vi "Write Channel.vi"(8 "error in (no error)":errorcluster, 10 "Channel":T1={"Coupling"=0, "Differential Input"=FALSE, "Direct-to-ADC"=FALSE, "Range"=2000, "Impedance"=50, "DC Offset"=0, "Filter"=0} {"Impedance" min=50 max=1000000 step=999950; "Coupling" items=["DC", "AC"]}, 11 "Initialize_card in":refnum<class "Control_card.lvclass">) -> (0 "error out":errorcluster, 3 "Initialize_card out":refnum<class "Control_card.lvclass">)   [LabVIEW 2015, in "Control_card.lvclass"]
uses:
  Control_card.lvclass
  Control_card.lvclass/Control_card.ctl
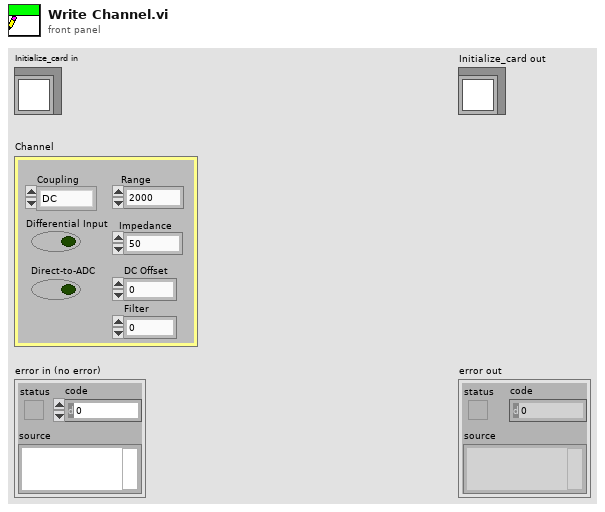
[diagram p1: front panel]
types:
  T1 = cluster{"Coupling":u16, "Differential Input":bool, "Direct-to-ADC":bool, "Range":u32, "Impedance":u32, "DC Offset":i32, "Filter":i32}
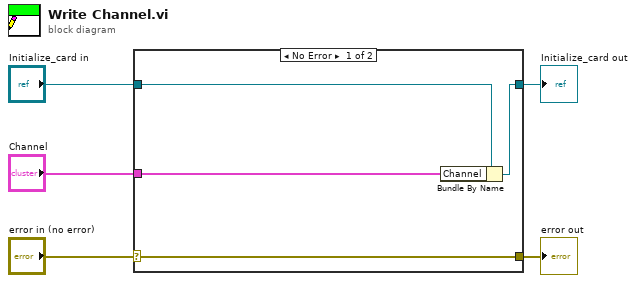
[diagram p0: block diagram]
diagram:
  n1 = case shown="No Error" "error in (no error)" {
    selector: "error in (no error)" -> [w9 w10]
    tunnel: [w9 w10] -> w4
    tunnel: [w7 w11] -> w2
    tunnel: "Initialize_card in" -> [w8 w11]
    tunnel: "Channel" -> [w6 _]
    frame No Error {
      n2 = Bundle By Name(cluster=w8, "Channel"=w6) -> (w7:refnum<class "Control_card.lvclass">)
    }
    frame Error {
    }
  }
  "error out" <- w4
  "Initialize_card out" <- w2
